vi "RTS Build Custom Header Array.vi"(8 "Error In":errorcluster, 9 "Listbox Item Names in":string[](array[string])=["System Date", "System Time", "Elapsed Time (sec)", "Elapsed Time (hrs)", "Voltage (V)", "RMS Current (Amps)", "Power (Watts)", "Watt Hours (Wh)", "Voltage Total Harmonic Distortion (%)", "Frequency (Hz)", "Apparent Power (VA)", "Power Factor", "TC 1", "TC 2", "TC 3", "TC 4", "TC 5", "TC 6", "TC 7", "TC 8", "TC 9", "TC 10", "TC 11", "TC 12", "TC 13", "TC 14", "TC 15", "TC 16", "TC 17", "TC 18", "TC 19", "TC 20", "TC 21", "TC 22", "TC 23", "TC 24", "TC 25", "TC 26", "TC 27", "TC 28", "TC 29", "TC 30", "AUX 1", "AUX 2", "CAL CL", "Room Setpoint Temperature", "Room Setpoint Humidity", "Room Temperature (°F)", "Room Humidity (%)", "Door Enable", "Room Setpoint Cool Temperature", "Room Setpoint Dehumidification Temperature", "Supply Temperature (°F)", "Cool Temperature (°F)", "Dehumidification Temperature (°F)", "Glycol Temperature (°F)", "Heat Rate (%)", "Steam Rate (%)", "Cool Rate (%)", "Dehumidification Rate (%)", "Room Status", "Room Dry P", "Room Dry I", "Room Humidity P", "Room Humidity I", "Room Heat P", "Room Heat I", "Room Cool Temperature P", "Room Cool Temperature I", "Room Dehumidification Temperature P", "Room Dehumidification Temperature I", "Voltage Setpoint 1", "60 Hz Power", "50 Hz Power", "120V Range", "240V Range", "Ground Line", "Ground Neutral", "Measure Ground Leakage Current", "Room OK", "S1 Freezer Relay", "S1 Cab Relay", "S1 Slide Relay", "Recording Data", "CVS Location", "Point Location"], 10 "Full Item Names":string[](array[string])=["System Date", "System Time", "Elapsed Time (sec)", "Elapsed Time (hrs)", "Voltage (V)", "RMS Current (Amps)", "Power (Watts)", "Watt Hours (Wh)", "Voltage Total Harmonic Distortion (%)", "Frequency (Hz)", "Apparent Power (VA)", "Power Factor", "TC 1", "TC 2", "TC 3", "TC 4", "TC 5", "TC 6", "TC 7", "TC 8", "TC 9", "TC 10", "TC 11", "TC 12", "TC 13", "TC 14", "TC 15", "TC 16", "TC 17", "TC 18", "TC 19", "TC 20", "TC 21", "TC 22", "TC 23", "TC 24", "TC 25", "TC 26", "TC 27", "TC 28", "TC 29", "TC 30", "AUX 1", "AUX 2", "CAL CL", "Room Setpoint Temperature", "Room Setpoint Humidity", "Room Temperature (°F)", "Room Humidity (%)", "Door Enable", "Room Setpoint Cool Temperature", "Room Setpoint Dehumidification Temperature", "Supply Temperature (°F)", "Cool Temperature (°F)", "Dehumidification Temperature (°F)", "Glycol Temperature (°F)", "Heat Rate (%)", "Steam Rate (%)", "Cool Rate (%)", "Dehumidification Rate (%)", "Room Status", "Room Dry P", "Room Dry I", "Room Humidity P", "Room Humidity I", "Room Heat P", "Room Heat I", "Room Cool Temperature P", "Room Cool Temperature I", "Room Dehumidification Temperature P", "Room Dehumidification Temperature I", "Voltage Setpoint 1", "60 Hz Power", "50 Hz Power", "120V Range", "240V Range", "Ground Line", "Ground Neutral", "Measure Ground Leakage Current", "Room OK", "S1 Freezer Relay", "S1 Cab Relay", "S1 Slide Relay", "Recording Data", "CVS Location", "Point Location"], 11 "All Data in":dbl[][](array[numeric])=[[3600091001.703, 12.0, 0.0, 0.0, 115.113976, 0.726104, 73.792992, 3453.956435, 3.4, 59.980007, 83.58474, 0.882852, 7.91, 6.92, 6.4, 327.67, 327.67, 327.67, 327.67, 327.67, 327.67, 327.67, 40.47, 39.09, 39.23, 327.67, 327.67, 327.67, 327.67, 327.67, 327.67, 327.67, 327.67, 327.67, 327.67, 69.95, 327.67, 327.67, 70.08, 327.67, 32767.0, 32767.0, 0.0, 0.0, 1.988, 70.0, 35.0, 69.85, 37.15, 1.0, 55.0, 48.0, 67.6, 55.36, 47.89, 0.0, 38.03, 0.09, 30.61, 7.12, 0.0, 200.0, 15000.0, 400.0, 15000.0, 1000.0, 2000.0, 500.0, 6000.0, 500.0, 6000.0, 115.0, 1.0, 0.0, 1.0, 0.0, 0.0, 1.0, 0.0, 0.0, 0.0, 0.0, 0.0, 0.0, 0.0, 0.0], [3600091002.724, 12.0, 0.0, 0.0, 115.113976, 0.732625, 74.150955, 3453.978342, 3.4, 59.981895, 84.335365, 0.879239, 7.91, 6.92, 6.4, 327.67, 327.67, 327.67, 327.67, 327.67, 327.67, 327.67, 40.47, 39.09, 39.23, 327.67, 327.67, 327.67, 327.67, 327.67, 327.67, 327.67, 327.67, 327.67, 327.67, 69.95, 327.67, 327.67, 70.08, 327.67, 32767.0, 32767.0, 0.001, 0.0, 1.988, 70.0, 35.0, 69.85, 37.15, 1.0, 55.0, 48.0, 67.6, 55.36, 47.89, 0.0, 38.03, 0.09, 30.61, 7.12, 0.0, 200.0, 15000.0, 400.0, 15000.0, 1000.0, 2000.0, 500.0, 6000.0, 500.0, 6000.0, 115.0, 1.0, 0.0, 1.0, 0.0, 0.0, 1.0, 0.0, 0.0, 0.0, 0.0, 0.0, 0.0, 0.0, 0.0], [3600091003.749, 12.0, 0.0, 0.0, 115.094734, 0.72875, 73.917732, 3454.000256, 3.4, 59.980373, 84.227455, 0.878872, 7.88, 6.92, 6.4, 327.67, 327.67, 327.67, 327.67, 327.67, 327.67, 327.67, 40.47, 39.09, 39.23, 327.67, 327.67, 327.67, 327.67, 327.67, 327.67, 327.67, 327.67, 327.67, 327.67, 70.0, 327.67, 327.67, 70.14, 327.67, 32767.0, 32767.0, 0.001, 0.0, 1.988, 70.0, 35.0, 69.85, 37.15, 1.0, 55.0, 48.0, 67.6, 55.36, 47.89, 0.0, 38.03, 0.09, 30.61, 7.12, 0.0, 200.0, 15000.0, 400.0, 15000.0, 1000.0, 2000.0, 500.0, 6000.0, 500.0, 6000.0, 115.0, 1.0, 0.0, 1.0, 0.0, 0.0, 1.0, 0.0, 0.0, 0.0, 0.0, 0.0, 0.0, 0.0, 0.0], [3600091004.771, 12.0, 0.0, 0.0, 115.123596, 0.731687, 73.960884, 3454.019387, 3.2, 59.983654, 84.234489, 0.878036, 7.88, 6.92, 6.4, 327.67, 327.67, 327.67, 327.67, 327.67, 327.67, 327.67, 40.47, 39.09, 39.23, 327.67, 327.67, 327.67, 327.67, 327.67, 327.67, 327.67, 327.67, 327.67, 327.67, 70.0, 327.67, 327.67, 70.14, 327.67, 32767.0, 32767.0, 0.001, 0.0, 1.987, 70.0, 35.0, 69.85, 37.15, 1.0, 55.0, 48.0, 67.6, 55.36, 47.89, 0.0, 38.02, 0.09, 30.61, 7.12, 0.0, 200.0, 15000.0, 400.0, 15000.0, 1000.0, 2000.0, 500.0, 6000.0, 500.0, 6000.0, 115.0, 1.0, 0.0, 1.0, 0.0, 0.0, 1.0, 0.0, 0.0, 0.0, 0.0, 0.0, 0.0, 0.0, 0.0], [3600091005.799, 12.0, 0.0, 0.0, 115.113976, 0.72825, 73.662361, 3454.041219, 3.4, 59.985176, 83.831749, 0.878693, 7.88, 6.92, 6.4, 327.67, 327.67, 327.67, 327.67, 327.67, 327.67, 327.67, 40.44, 39.04, 39.23, 327.67, 327.67, 327.67, 327.67, 327.67, 327.67, 327.67, 327.67, 327.67, 327.67, 70.0, 327.67, 327.67, 70.14, 327.67, 32767.0, 32767.0, 0.001, 0.0, 1.987, 70.0, 35.0, 69.85, 37.15, 1.0, 55.0, 48.0, 67.6, 55.36, 47.89, 0.0, 38.02, 0.09, 30.61, 7.12, 0.0, 200.0, 15000.0, 400.0, 15000.0, 1000.0, 2000.0, 500.0, 6000.0, 500.0, 6000.0, 115.0, 1.0, 0.0, 1.0, 0.0, 0.0, 1.0, 0.0, 0.0, 0.0, 0.0, 0.0, 0.0, 0.0, 0.0], [3600091006.815, 12.0, 0.0, 0.0, 115.123596, 0.725771, 73.487831, 3454.063036, 3.4, 59.986942, 83.553345, 0.879532, 7.88, 6.92, 6.4, 327.67, 327.67, 327.67, 327.67, 327.67, 327.67, 327.67, 40.44, 39.04, 39.23, 327.67, 327.67, 327.67, 327.67, 327.67, 327.67, 327.67, 327.67, 327.67, 327.67, 70.0, 327.67, 327.67, 70.14, 327.67, 32767.0, 32767.0, 0.001, 0.0, 1.988, 70.0, 35.0, 69.85, 37.15, 1.0, 55.0, 48.0, 67.6, 55.36, 47.89, 0.0, 38.02, 0.08, 30.61, 7.12, 0.0, 200.0, 15000.0, 400.0, 15000.0, 1000.0, 2000.0, 500.0, 6000.0, 500.0, 6000.0, 115.0, 1.0, 0.0, 1.0, 0.0, 0.0, 1.0, 0.0, 0.0, 0.0, 0.0, 0.0, 0.0, 0.0, 0.0], [3600091007.834, 12.0, 0.0, 0.0, 115.104355, 0.728729, 73.744789, 3454.082127, 3.4, 59.984016, 83.879898, 0.879171, 7.88, 6.92, 6.4, 327.67, 327.67, 327.67, 327.67, 327.67, 327.67, 327.67, 40.44, 39.04, 39.23, 327.67, 327.67, 327.67, 327.67, 327.67, 327.67, 327.67, 327.67, 327.67, 327.67, 70.0, 327.67, 327.67, 70.14, 327.67, 32767.0, 32767.0, 0.001, 0.0, 1.988, 70.0, 35.0, 69.85, 37.15, 1.0, 55.0, 48.0, 67.6, 55.36, 47.89, 0.0, 38.02, 0.08, 30.61, 7.12, 0.0, 200.0, 15000.0, 400.0, 15000.0, 1000.0, 2000.0, 500.0, 6000.0, 500.0, 6000.0, 115.0, 1.0, 0.0, 1.0, 0.0, 0.0, 1.0, 0.0, 0.0, 0.0, 0.0, 0.0, 0.0, 0.0, 0.0], [3600091008.851, 12.0, 0.0, 0.0, 115.123596, 0.726167, 73.607307, 3454.103967, 3.3, 59.985229, 83.598915, 0.880482, 7.88, 6.92, 6.4, 327.67, 327.67, 327.67, 327.67, 327.67, 327.67, 327.67, 40.44, 39.04, 39.23, 327.67, 327.67, 327.67, 327.67, 327.67, 327.67, 327.67, 327.67, 327.67, 327.67, 70.0, 327.67, 327.67, 70.14, 327.67, 32767.0, 32767.0, 0.001, 0.001, 1.988, 70.0, 35.0, 69.85, 37.15, 1.0, 55.0, 48.0, 67.6, 55.36, 47.89, 0.0, 38.02, 0.08, 30.61, 7.12, 0.0, 200.0, 15000.0, 400.0, 15000.0, 1000.0, 2000.0, 500.0, 6000.0, 500.0, 6000.0, 115.0, 1.0, 0.0, 1.0, 0.0, 0.0, 1.0, 0.0, 0.0, 0.0, 0.0, 0.0, 0.0, 0.0, 0.0], [3600091009.874, 12.0, 0.0, 0.0, 115.113976, 0.728542, 73.781647, 3454.123084, 3.4, 59.985569, 83.865326, 0.879763, 7.88, 6.87, 6.4, 327.67, 327.67, 327.67, 327.67, 327.67, 327.67, 327.67, 40.47, 39.04, 39.23, 327.67, 327.67, 327.67, 327.67, 327.67, 327.67, 327.67, 327.67, 327.67, 327.67, 70.0, 327.67, 327.67, 70.14, 327.67, 32767.0, 32767.0, 0.001, 0.001, 1.988, 70.0, 35.0, 69.85, 37.15, 1.0, 55.0, 48.0, 67.6, 55.36, 47.89, 0.0, 38.01, 0.08, 30.61, 7.12, 0.0, 200.0, 15000.0, 400.0, 15000.0, 1000.0, 2000.0, 500.0, 6000.0, 500.0, 6000.0, 115.0, 1.0, 0.0, 1.0, 0.0, 0.0, 1.0, 0.0, 0.0, 0.0, 0.0, 0.0, 0.0, 0.0, 0.0], [3600091010.892, 12.0, 0.0, 0.0, 115.104355, 0.725438, 73.578506, 3454.144929, 3.3, 59.984901, 83.501015, 0.881169, 7.88, 6.87, 6.4, 327.67, 327.67, 327.67, 327.67, 327.67, 327.67, 327.67, 40.47, 39.04, 39.23, 327.67, 327.67, 327.67, 327.67, 327.67, 327.67, 327.67, 327.67, 327.67, 327.67, 70.0, 327.67, 327.67, 70.14, 327.67, 32767.0, 32767.0, 0.001, 0.001, 1.988, 70.0, 35.0, 69.85, 37.15, 1.0, 55.0, 48.0, 67.6, 55.36, 47.89, 0.0, 38.01, 0.08, 30.61, 7.12, 0.0, 200.0, 15000.0, 400.0, 15000.0, 1000.0, 2000.0, 500.0, 6000.0, 500.0, 6000.0, 115.0, 1.0, 0.0, 1.0, 0.0, 0.0, 1.0, 0.0, 0.0, 0.0, 0.0, 0.0, 0.0, 0.0, 0.0], [3600091011.915, 12.0, 0.0, 0.0, 115.104355, 0.722, 73.502365, 3454.16674, 3.4, 59.98167, 83.105339, 0.884448, 7.83, 6.87, 6.4, 327.67, 327.67, 327.67, 327.67, 327.67, 327.67, 327.67, 40.44, 39.04, 39.23, 327.67, 327.67, 327.67, 327.67, 327.67, 327.67, 327.67, 327.67, 327.67, 327.67, 69.92, 327.67, 327.67, 70.08, 327.67, 32767.0, 32767.0, 0.001, 0.001, 1.988, 70.0, 35.0, 69.85, 37.15, 1.0, 55.0, 48.0, 67.6, 55.36, 47.89, 0.0, 38.01, 0.08, 30.61, 7.12, 0.0, 200.0, 15000.0, 400.0, 15000.0, 1000.0, 2000.0, 500.0, 6000.0, 500.0, 6000.0, 115.0, 1.0, 0.0, 1.0, 0.0, 0.0, 1.0, 0.0, 0.0, 0.0, 0.0, 0.0, 0.0, 0.0, 0.0], [3600091012.934, 12.0, 0.0, 0.0, 115.094727, 0.723542, 73.421265, 3454.185795, 3.4, 59.981655, 83.275833, 0.881664, 7.83, 6.87, 6.4, 327.67, 327.67, 327.67, 327.67, 327.67, 327.67, 327.67, 40.44, 39.04, 39.23, 327.67, 327.67, 327.67, 327.67, 327.67, 327.67, 327.67, 327.67, 327.67, 327.67, 69.92, 327.67, 327.67, 70.08, 327.67, 32767.0, 32767.0, 0.001, 0.0, 1.988, 70.0, 35.0, 69.85, 37.15, 1.0, 55.0, 48.0, 67.6, 55.36, 47.89, 0.0, 38.01, 0.07, 30.62, 7.12, 0.0, 200.0, 15000.0, 400.0, 15000.0, 1000.0, 2000.0, 500.0, 6000.0, 500.0, 6000.0, 115.0, 1.0, 0.0, 1.0, 0.0, 0.0, 1.0, 0.0, 0.0, 0.0, 0.0, 0.0, 0.0, 0.0, 0.0], [3600091013.956, 12.0, 0.0, 0.0, 115.113976, 0.721937, 73.541336, 3454.207582, 3.3, 59.98288, 83.105095, 0.88492, 7.83, 6.87, 6.4, 327.67, 327.67, 327.67, 327.67, 327.67, 327.67, 327.67, 40.44, 39.04, 39.23, 327.67, 327.67, 327.67, 327.67, 327.67, 327.67, 327.67, 327.67, 327.67, 327.67, 70.0, 327.67, 327.67, 70.14, 327.67, 32767.0, 32767.0, 0.001, 0.0, 1.988, 70.0, 35.0, 69.85, 37.15, 1.0, 55.0, 48.0, 67.33, 55.36, 47.89, 0.0, 38.0, 0.07, 30.62, 7.12, 0.0, 200.0, 15000.0, 400.0, 15000.0, 1000.0, 2000.0, 500.0, 6000.0, 500.0, 6000.0, 115.0, 1.0, 0.0, 1.0, 0.0, 0.0, 1.0, 0.0, 0.0, 0.0, 0.0, 0.0, 0.0, 0.0, 0.0], [3600091014.973, 12.0, 0.0, 0.0, 115.133224, 0.725083, 73.722015, 3454.229415, 3.4, 59.983387, 83.481186, 0.883097, 7.83, 6.87, 6.4, 327.67, 327.67, 327.67, 327.67, 327.67, 327.67, 327.67, 40.44, 39.04, 39.23, 327.67, 327.67, 327.67, 327.67, 327.67, 327.67, 327.67, 327.67, 327.67, 327.67, 70.0, 327.67, 327.67, 70.14, 327.67, 32767.0, 32767.0, 0.001, 0.0, 1.988, 70.0, 35.0, 69.85, 37.15, 1.0, 55.0, 48.0, 67.33, 55.36, 47.89, 0.0, 39.04, 0.07, 30.62, 7.12, 0.0, 200.0, 15000.0, 400.0, 15000.0, 1000.0, 2000.0, 500.0, 6000.0, 500.0, 6000.0, 115.0, 1.0, 0.0, 1.0, 0.0, 0.0, 1.0, 0.0, 0.0, 0.0, 0.0, 0.0, 0.0, 0.0, 0.0], [3600091015.997, 12.0, 0.0, 0.0, 115.094727, 0.722229, 73.60537, 3454.24855, 3.3, 59.983395, 83.124771, 0.885481, 7.83, 6.87, 6.4, 327.67, 327.67, 327.67, 327.67, 327.67, 327.67, 327.67, 40.44, 39.04, 39.23, 327.67, 327.67, 327.67, 327.67, 327.67, 327.67, 327.67, 327.67, 327.67, 327.67, 70.0, 327.67, 327.67, 70.14, 327.67, 32767.0, 32767.0, 0.001, 0.0, 1.988, 70.0, 35.0, 69.85, 37.15, 1.0, 55.0, 48.0, 67.33, 55.36, 47.89, 0.0, 39.04, 0.07, 30.62, 7.12, 0.0, 200.0, 15000.0, 400.0, 15000.0, 1000.0, 2000.0, 500.0, 6000.0, 500.0, 6000.0, 115.0, 1.0, 0.0, 1.0, 0.0, 0.0, 1.0, 0.0, 0.0, 0.0, 0.0, 0.0, 0.0, 0.0, 0.0], [3600091017.018, 12.0, 0.0, 0.0, 115.142845, 0.728646, 73.968193, 3454.270419, 3.2, 59.984619, 83.898354, 0.881641, 7.83, 6.87, 6.35, 327.67, 327.67, 327.67, 327.67, 327.67, 327.67, 327.67, 40.44, 39.04, 39.23, 327.67, 327.67, 327.67, 327.67, 327.67, 327.67, 327.67, 327.67, 327.67, 327.67, 70.0, 327.67, 327.67, 70.14, 327.67, 32767.0, 32767.0, 0.001, 0.001, 1.988, 70.0, 35.0, 69.85, 37.15, 1.0, 55.0, 48.0, 67.33, 55.36, 47.89, 0.0, 39.04, 0.07, 30.62, 7.12, 0.0, 200.0, 15000.0, 400.0, 15000.0, 1000.0, 2000.0, 500.0, 6000.0, 500.0, 6000.0, 115.0, 1.0, 0.0, 1.0, 0.0, 0.0, 1.0, 0.0, 0.0, 0.0, 0.0, 0.0, 0.0, 0.0, 0.0], [3600091018.039, 12.0, 0.0, 0.0, 115.104355, 0.73125, 73.90947, 3454.292285, 3.3, 59.98568, 84.170059, 0.878097, 7.83, 6.87, 6.35, 327.67, 327.67, 327.67, 327.67, 327.67, 327.67, 327.67, 40.44, 39.04, 39.23, 327.67, 327.67, 327.67, 327.67, 327.67, 327.67, 327.67, 327.67, 327.67, 327.67, 69.95, 327.67, 327.67, 70.08, 327.67, 32767.0, 32767.0, 0.001, 0.001, 1.988, 70.0, 35.0, 69.85, 37.15, 1.0, 55.0, 48.0, 67.33, 55.36, 47.89, 0.0, 39.05, 0.07, 30.62, 7.12, 0.0, 200.0, 15000.0, 400.0, 15000.0, 1000.0, 2000.0, 500.0, 6000.0, 500.0, 6000.0, 115.0, 1.0, 0.0, 1.0, 0.0, 0.0, 1.0, 0.0, 0.0, 0.0, 0.0, 0.0, 0.0, 0.0, 0.0], [3600091019.059, 12.0, 0.0, 0.0, 115.104355, 0.727896, 73.668884, 3454.311388, 3.3, 59.986122, 83.783981, 0.879272, 7.83, 6.87, 6.4, 327.67, 327.67, 327.67, 327.67, 327.67, 327.67, 327.67, 40.44, 39.04, 39.23, 327.67, 327.67, 327.67, 327.67, 327.67, 327.67, 327.67, 327.67, 327.67, 327.67, 69.95, 327.67, 327.67, 70.08, 327.67, 32767.0, 32767.0, 0.001, 0.001, 1.988, 70.0, 35.0, 69.85, 37.15, 1.0, 55.0, 48.0, 67.33, 55.36, 47.89, 0.0, 39.05, 0.07, 30.62, 7.12, 0.0, 200.0, 15000.0, 400.0, 15000.0, 1000.0, 2000.0, 500.0, 6000.0, 500.0, 6000.0, 115.0, 1.0, 0.0, 1.0, 0.0, 0.0, 1.0, 0.0, 0.0, 0.0, 0.0, 0.0, 0.0, 0.0, 0.0], [3600091020.076, 12.0, 0.0, 0.0, 115.113976, 0.729708, 73.698441, 3454.333193, 3.3, 59.986202, 83.999626, 0.877366, 7.83, 6.87, 6.4, 327.67, 327.67, 327.67, 327.67, 327.67, 327.67, 327.67, 40.44, 39.04, 39.23, 327.67, 327.67, 327.67, 327.67, 327.67, 327.67, 327.67, 327.67, 327.67, 327.67, 69.95, 327.67, 327.67, 70.08, 327.67, 32767.0, 32767.0, 0.001, 0.001, 1.988, 70.0, 35.0, 69.85, 37.15, 1.0, 55.0, 48.0, 67.33, 55.36, 47.89, 0.0, 39.05, 0.06, 30.62, 7.12, 0.0, 200.0, 15000.0, 400.0, 15000.0, 1000.0, 2000.0, 500.0, 6000.0, 500.0, 6000.0, 115.0, 1.0, 0.0, 1.0, 0.0, 0.0, 1.0, 0.0, 0.0, 0.0, 0.0, 0.0, 0.0, 0.0, 0.0]] format="%.6f") -> (0 "Error Out":errorcluster, 1 "Listbox Item Names out":string[](array[string]), 2 "Parsed Array":dbl[][](array[numeric]), 3 "Time Data":dbl[](array[numeric]), 5 "Index Locations":i32[](array[numeric]))   [LabVIEW 2016]
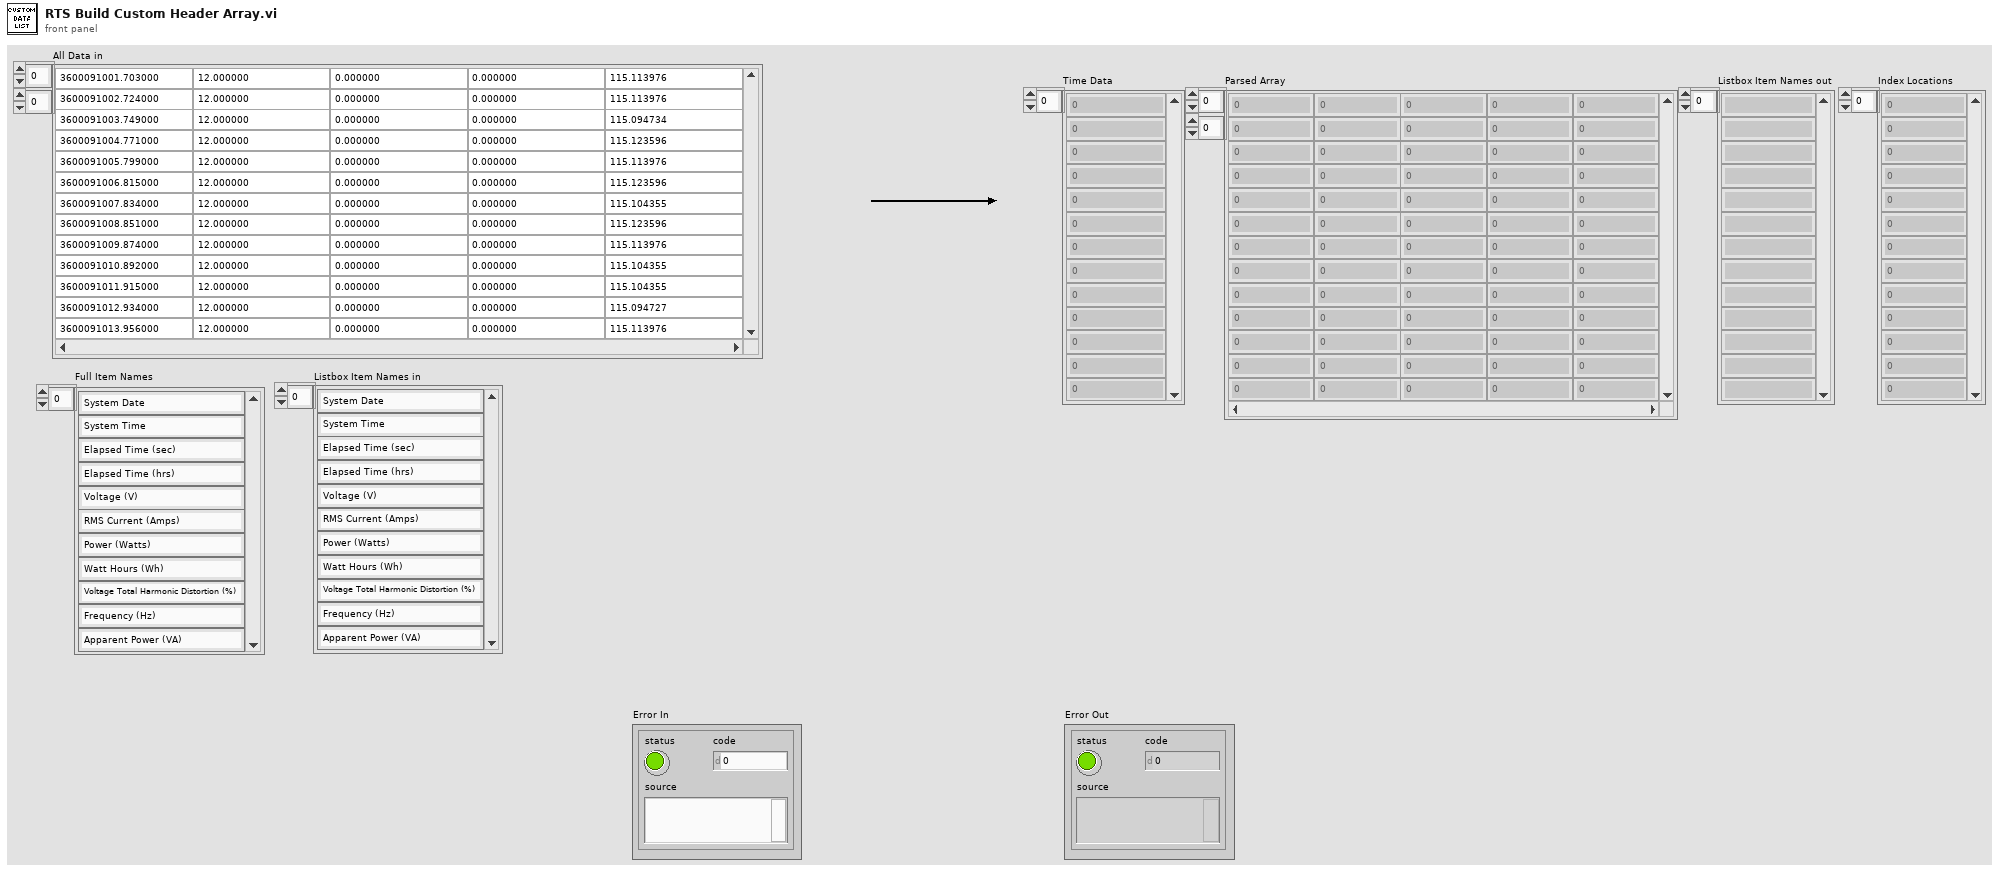
[diagram p1: front panel]
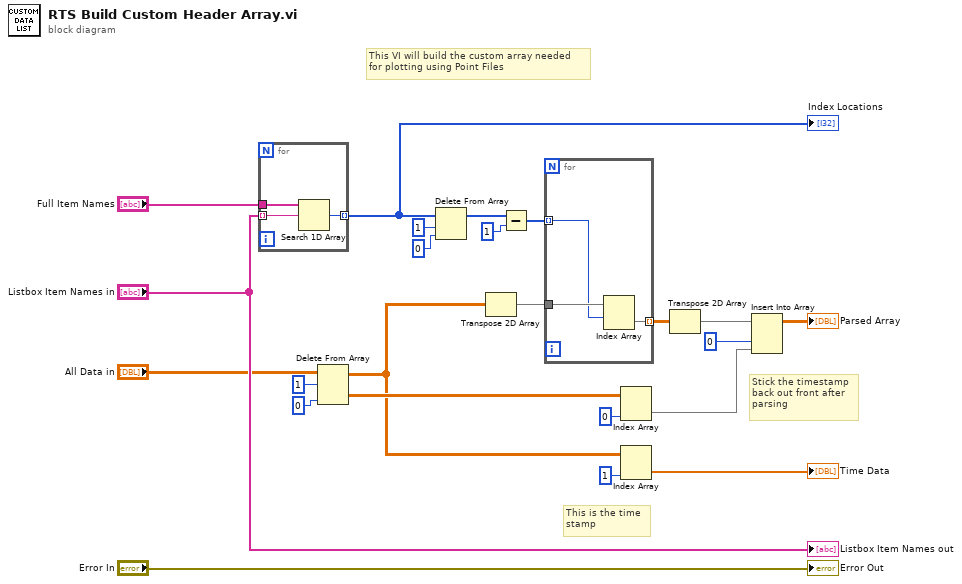
[diagram p0: block diagram]
diagram:
  # "This VI will build the custom array needed\nfor plotting using Point Files"
  # "Stick the timestamp\nback out front after\nparsing"
  # "This is the time \nstamp"
  n1 = for {
    tunnel: "Full Item Names" -> [w26]
    tunnel: "Listbox Item Names in" -> [w25] mode=indexing
    tunnel: [w24] -> w7 mode=indexing
    n2 = Search 1D Array(1D array=w26, element=w25) -> (index of element=w24:i32)  [unwired: 1 in]
  }
  "Index Locations" <- w7
  n3 = Delete From Array(array="All Data in", length=1, index (col)=0 ("index (row)")) -> (deleted portion=w4:dbl[][], array with subset deleted=w1:dbl[][])  [unwired: 1 in]
  n4 = Delete From Array(array=w7, length=1, index=0) -> (array with subset deleted=w18:i32[])  [unwired: 1 out]
  n5 = Transpose 2D Array(2D array=w1) -> (transposed array=w16:dbl[][])
  n6 = Subtract(x=w18, y=1 ("length")) -> (x-y=w19:i32[])
  n7 = for {
    tunnel: w19 -> [w28] mode=indexing
    tunnel: w16 -> [w29]
    tunnel: [w27] -> w17 mode=indexing
    n8 = Index Array(array=w29, index (row)=w28) -> (element=w27:dbl[])  [unwired: 1 in]
  }
  n9 = Index Array(array=w4, index (col)=0 ("disabled index (col)")) -> (element=w20:dbl[])  [unwired: 1 in]
  n10 = Index Array(array=w1, index (col)=1 ("disabled index (col)")) -> (element=→"Time Data":dbl[])  [unwired: 1 in]
  n11 = Transpose 2D Array(2D array=w17) -> (transposed array=w23:dbl[][])
  n12 = Insert Into Array(array=w23, index (col)=0 ("disabled index (col)"), new element=w20) -> (→"Parsed Array":dbl[][])  [unwired: 1 in]
  "Listbox Item Names out" <- "Listbox Item Names in"
  "Error Out" <- "Error In"
